vi "HEWH RLT Cutout Delay Message.vi"(8 "error in (no error)":errorcluster, 10 "Heat Source ON (1=ON)":bool, 11 "Start Draw":bool) -> (0 "error out":errorcluster)   [LabVIEW 2023]
uses:
  Utility/Custom Pallet Controls/Custom Pallet String.ctl
  Utility/Type Definitions/UTILITY Notifier.ctl
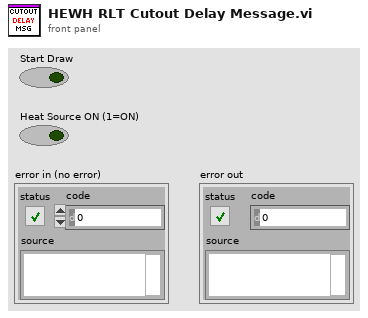
[diagram p1: front panel]
types:
  T1 = typedef "UTILITY Notifier.ctl" = enum16{"Set", "Read", "Release Ref"}
  T2 = typedef "Custom Pallet String.ctl" = string
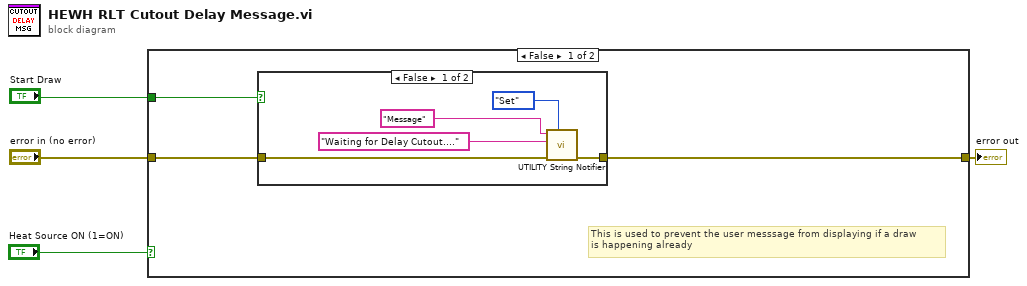
[diagram p0: block diagram]
diagram:
  n1 = case shown="False" "Heat Source ON (1=ON)" {
    tunnel: "error in (no error)" -> [w7 w14]
    tunnel: [w6 w14] -> w2
    tunnel: "Start Draw" -> [w5 _]
    frame False {
      # "This is used to prevent the user messsage from displaying if a draw \nis happening already"
      n2 = case shown="False" w5 {
        tunnel: w7 -> [w10 w13]
        tunnel: [w9 w13] -> w6
        frame False {
          n3 = call "UTILITY String Notifier.vi"("Status"=UTILITY_Notifier."Set", "error in (no error)"=w10, "Set Status"=T2 "Waiting for Delay Cutout...." ("Message"), "name (unnamed)"="Message") -> ("error out"=w9:errorcluster)  [unwired: 6 in, 1 out]
        }
        frame True {
        }
      }
    }
    frame True {
    }
  }
  "error out" <- w2
